vi "Initialize Folder Structure.vi"(8 "error in (no error)":errorcluster, 11 "Project in":refnum<class "Project.lvclass">) -> (0 "error out":errorcluster, 3 "Project out":refnum<class "Project.lvclass">)   [LabVIEW 2025, in "Project.lvclass"]
doc: "Add project folder for dynamically generated project items."
uses:
  Project.lvclass
  Project.lvclass/Project.ctl
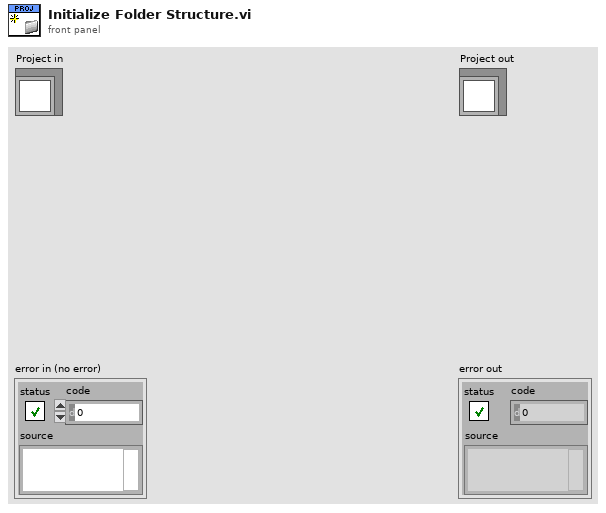
[diagram p1: front panel]
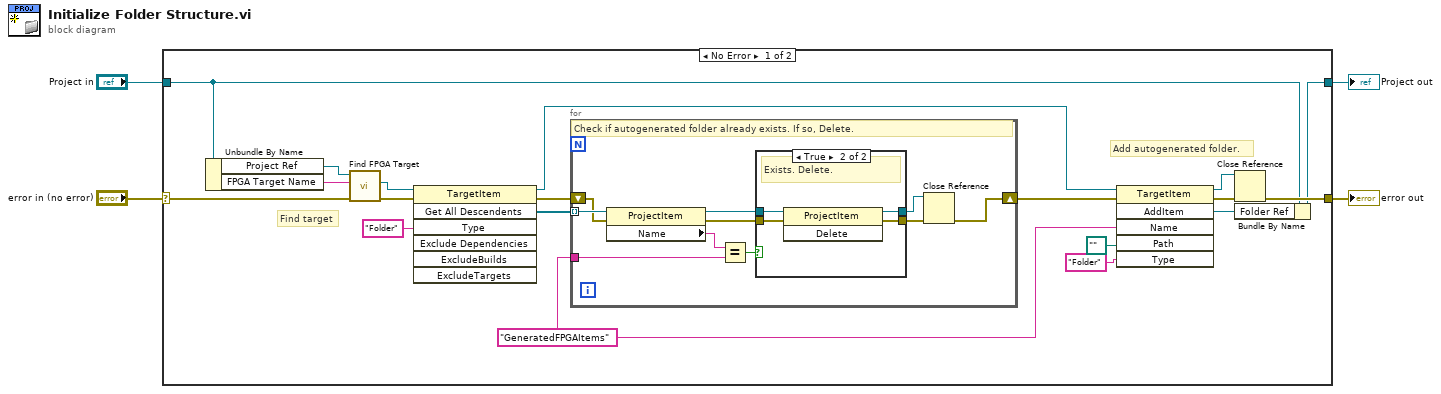
[diagram p0: block diagram]
diagram:
  n1 = case shown="No Error" "error in (no error)" {
    selector: "error in (no error)" -> [w6 w41]
    tunnel: [w12 w41] -> w3
    tunnel: [w8 w40] -> w1
    tunnel: "Project in" -> [w9 w40]
    frame No Error {
      w15 = "GeneratedFPGAItems" ("Name")
      # "Find target"
      # "Add autogenerated folder."
      n2 = Unbundle By Name(w9) -> ("Project Ref"=w7:refnum<vi>, "FPGA Target Name"=w11:string)
      n3 = call "Find FPGA Target.vi"("error in (no error)"=w6, "FPGA Target Name"=w11, "Project in"=w7) -> ("error out"=w17:errorcluster, "TargetItem out"=w5:refnum<vi>)  [unwired: 6 in, 1 out]
      n4 = invoke class="TargetItem" method="Get All Descendents"(reference=w5, error in=w17, "Type"="Folder") -> (reference out=w16:refnum<vi>, error out=w18:errorcluster, "All Descendents"=w19:refnum<vi>[])  [unwired: 4 in, 4 out]
      n5 = for {
        tunnel: w19 -> [w33] mode=indexing
        shift-right: [w24] -> w22
        shift-left: w18 -> [w32]
        tunnel: w15 -> [w30]
        # "Check if autogenerated folder already exists. If so, Delete."
        n6 = property class="ProjectItem"(reference=w33, error in=w32) -> (reference out=w29:refnum<vi>, error out=w28:errorcluster, "Name"=w31:string)
        n7 = Equal?(x=w31, y=w30) -> (x = y?=w27:bool)
        n8 = case shown="True" w27 {
          tunnel: w29 -> [w34 w39]
          tunnel: w28 -> [w35 w38]
          tunnel: [w35 w37] -> w25
          tunnel: [w34 w36] -> w26
          frame False {
          }
          frame True {
            # "Exists. Delete."
            n9 = invoke class="ProjectItem" method="Delete"(reference=w39, error in=w38) -> (reference out=w36:refnum<vi>, error out=w37:errorcluster)  [unwired: 1 in, 1 out]
          }
        }
        n10 = Close Reference(reference=w26, error in (no error)=w25) -> (error out=w24:errorcluster)
      }
      n11 = invoke class="TargetItem" method="AddItem"(reference=w16, error in=w22, "Name"=w15, "Path"=path "", "Type"="Folder") -> (reference out=w14:refnum<vi>, error out=w13:errorcluster, "AddItem"=w10:refnum<vi>)  [unwired: 1 in, 3 out]
      n12 = Close Reference(reference=w14, error in (no error)=w13) -> (error out=w12:errorcluster)
      n13 = Bundle By Name(cluster=w9, "Folder Ref"=w10) -> (w8:refnum<class "Project.lvclass">)
    }
    frame Error {
    }
  }
  "error out" <- w3
  "Project out" <- w1
